vi "Probe_DB.vi"() -> ()   [LabVIEW 2019]
uses:
  <vilib>/drjdpowell/SQLite Library/SQL Connection/Open (path).vi
  <vilib>/drjdpowell/SQLite Library/SQL Connection/Open (string).vi
  <vilib>/AdvancedString/Path To Command Line String.vi
  <vilib>/drjdpowell/SQLite Library/SQL Connection/Execute SQL (No results).vi
  <vilib>/drjdpowell/SQLite Library/SQL Connection/Connection.lvclass
  <vilib>/drjdpowell/SQLite Library/SQLite.lvlib
panel:
  in  "Resistencia":i32
  in  "Corriente":dbl
  in  "Voltaje":dbl
  in  "Temperatura":dbl
  in  "Humedad":dbl
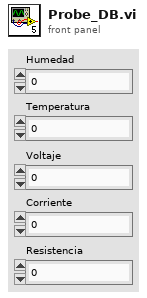
[diagram p1: front panel]
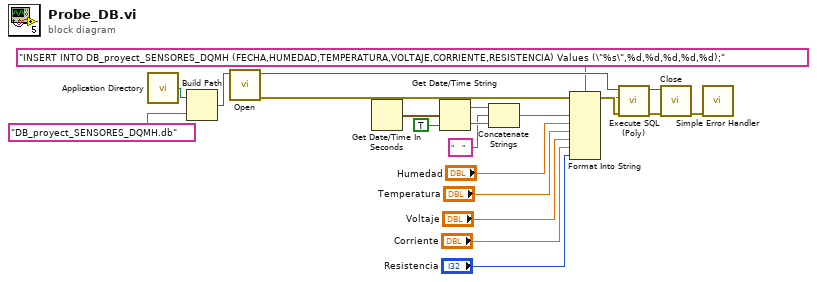
[diagram p0: block diagram]
diagram:
  n1 = call <vilib>:"Application Directory.vi"() -> ("Application Directory"=w16:path)
  n2 = Build Path(base path=w16, name or relative path="DB_proyect_SENSORES_DQMH.db") -> (appended path=w14:path)
  n3 = call-poly <vilib>:"Open.vi"("db file"=w14) -> ("error out"=w18:errorcluster, "SQLite Connection"=w21:refnum<class "Connection.lvclass">)  [unwired: 9 in]
  n4 = Get Date/Time In Seconds() -> (seconds since 1Jan1904=w6:timestamp)
  n5 = Get Date/Time String(seconds (now)=w6, want seconds? (F)=TRUE) -> (date string=w4:string, time string=w2:string)  [unwired: 1 in]
  n6 = Concatenate Strings(w4, "    " ("string"), w2) -> (w3:string)
  n7 = Format Into String(format string="INSERT INTO DB_proyect_SENSORES_DQMH (FECHA,HUMEDAD,TEMPERATURA,VOLTAJE,CORRIENTE,RESISTENCIA) Values (\"%s\",%d,%d,%d,%d,%d);", w3, "Humedad", "Temperatura", "Voltaje", "Corriente", "Resistencia") -> (resulting string=w13:string)  [unwired: 2 in, 1 out]
  n8 = call-poly <vilib>:"Execute SQL (Poly).vi"("error in (no error)"=w18, "SQL"=w13, "SQLite Connection in"=w21) -> ("error out"=w19:errorcluster, "SQLite Connection"=w20:refnum<class "Connection.lvclass">)  [unwired: 7 in]
  n9 = call-dynamic "Close.vi"("error in (no error)"=w19, "SQLite Connection in"=w20) -> ("error out"=w17:errorcluster)  [unwired: 9 in]
  n10 = call <vilib>:"Simple Error Handler.vi"("error in (no error)"=w17) -> ()  [unwired: 4 in, 5 out]
